vi "generate_DAC_voltages_V3_justMineZtrajectory.vi"(7 "focus mode?":bool, 8 "derived values":T1, 9 "scan specification":T4={"x amplitude"=0, "x resolution (pixels)"=0, "x offset fly-forward (iterations)"=0, "x offset fly-back (iterations)"=0, "y resolution (nr. of lines)"=0, "y step size"=0, "iterations per pixel"=0, "number of frames"=0, "y offset (pixels)"=0, "number of y-brake lines  (before y-fly-back)"=0, "number y-brake lines (after y-fly-back)"=0, "number of y-fly-back steps"=8, "lines per z step"=0, "number of z/intensity tuples"=0, "number of repetitions (volumes or planes)"=0, "z step size derived"=0, "choose the beginning of z scan"=FALSE, "number of frames (settings)"=0, "FPGA trajectory?"=FALSE}, 10 "counter cluster in":T2, 11 "resonant trigger":bool) -> (0 "acquire?":bool, 1 "fly-back acquisition phase?":bool, 2 "counter cluster out":T2, 3 "DAC voltages":T3 {"ch6" max=4095 step=1; "ch5" max=4095 step=1; "ch4" max=4095 step=1; "ch3" max=4095 step=1; "ch2" max=4095 step=1; "ch1" max=4095 step=1; "ch0" max=4095 step=1})   [LabVIEW 2010]
uses:
  scan_specification_cluster.ctl
  common_typedefs/DAC_voltage_cluster.ctl
  counter_cluster.ctl
  derived_values_cluster.ctl
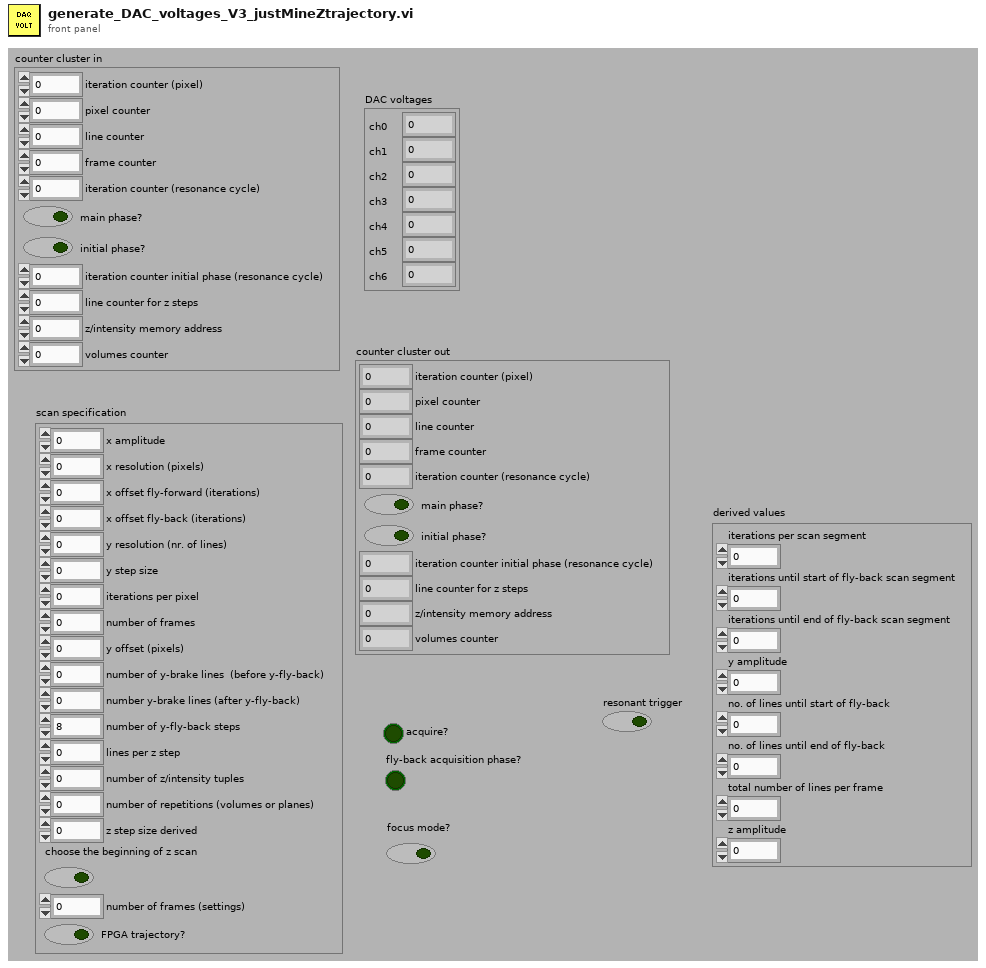
[diagram p1: front panel]
types:
  T1 = typedef "derived_values_cluster.ctl" = cluster{"iterations per scan segment":u16, "iterations until start of fly-back scan segment":u16, "iterations until end of fly-back scan segment":u16, "y amplitude":u16, "no. of lines until start of fly-back":u16, "no. of lines until end of fly-back":u16, "total number of lines per frame ":u16, "z amplitude":u16}
  T2 = typedef "counter_cluster.ctl" = cluster{"iteration counter (pixel)":u16, "pixel counter":u16, "line counter":u16, "frame counter":u16, "iteration counter (resonance cycle)":u16, "main phase?":bool, "initial phase?":bool, "iteration counter initial phase (resonance cycle)":u16, "line counter for z steps":u16, "z/intensity memory address":u32, "volumes counter":u16}
  T3 = typedef "DAC_voltage_cluster.ctl" = cluster{"ch0":u16, "ch1":i16, "ch2":i16, "ch3":u16, "ch4":u16, "ch5":u16, "ch6":u16}
  T4 = typedef "scan_specification_cluster.ctl" = cluster{"x amplitude":u16, "x resolution (pixels)":u16, "x offset fly-forward (iterations)":u16, "x offset fly-back (iterations)":u16, "y resolution (nr. of lines)":u16, "y step size":u16, "iterations per pixel":u16, "number of frames":i32, "y offset (pixels)":u16, "number of y-brake lines  (before y-fly-back)":u16, "number y-brake lines (after y-fly-back)":u16, "number of y-fly-back steps":u16, "lines per z step":u16, "number of z/intensity tuples":u16, "number of repetitions (volumes or planes)":i32, "z step size derived":u16, "choose the beginning of z scan":bool, "number of frames (settings)":i32, "FPGA trajectory?":bool}
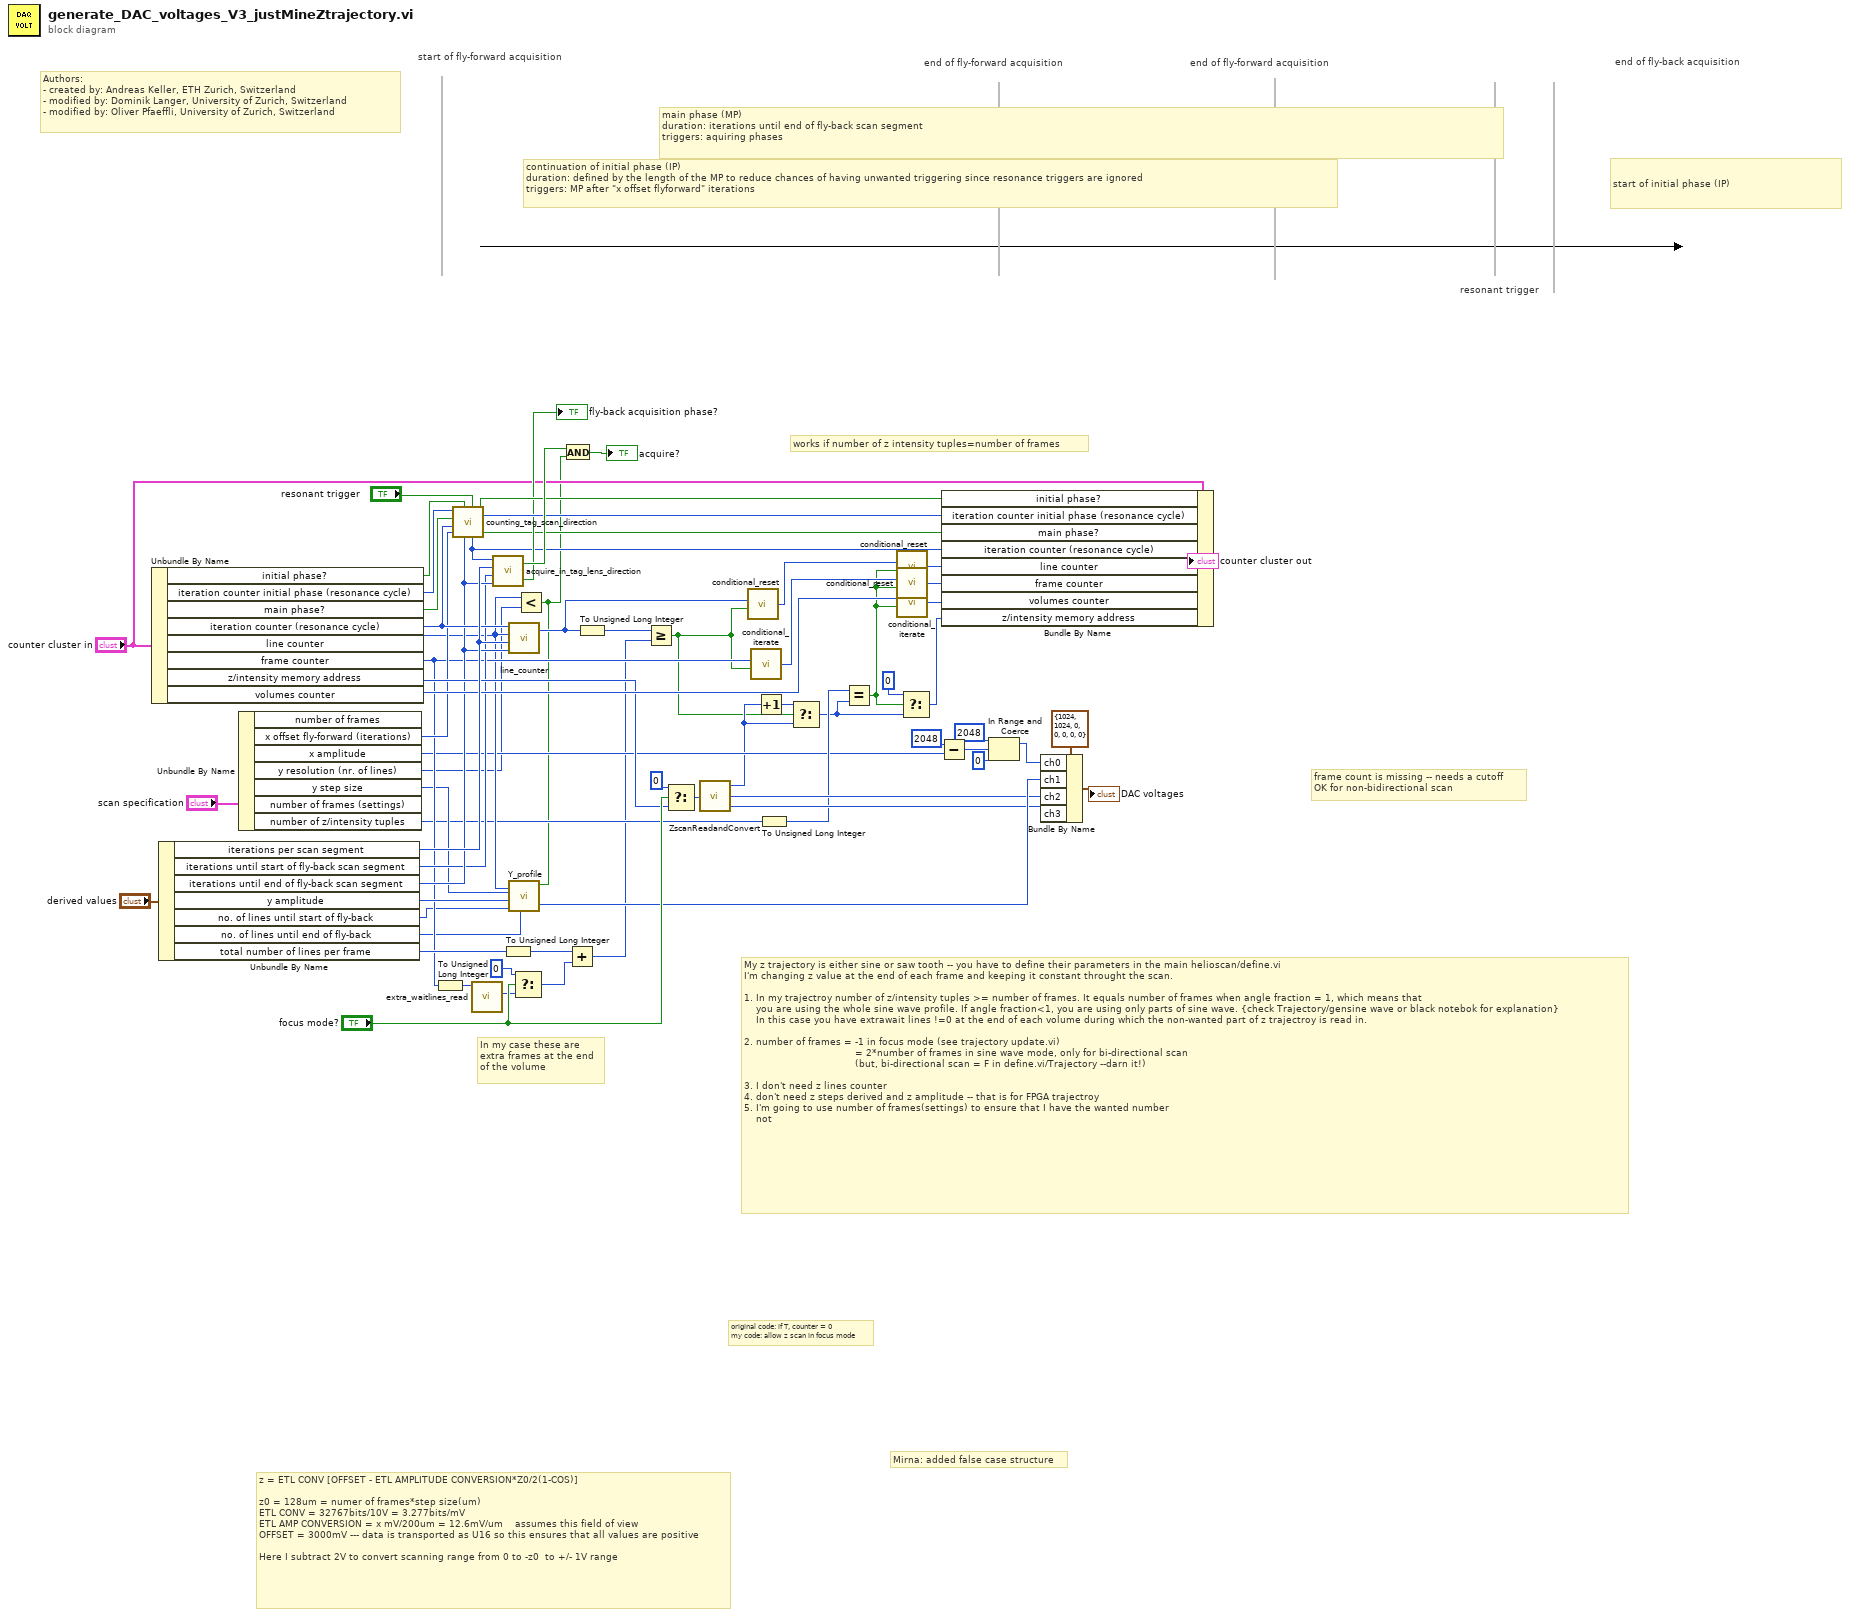
[diagram p0: block diagram]
diagram:
  # "works if number of z intensity tuples=number of frames"
  # "frame count is missing -- needs a cutoff\nOK for non-bidirectional scan"
  # "In my case these are \nextra frames at the end \nof the volume"
  # "My z trajectory is either sine or saw tooth -- you have to define their parameters in the main helioscan/define.vi\nI'm changing z value at the end of each frame and keeping it constant throught the scan.\n\n1. In my trajectroy number of z/intensity tuples >= number of frames. It equals number of frames when angle fraction = 1, which means that \n    you are using the whole sine wave profile. If angle fraction<1, you are using only parts of sine wave. {check Trajectory/gensine wave or black notebok for explanation}\n    In this case you have extrawait lines !=0 at the end of each volume during which the non-wanted part of z trajectroy is read in.\n   \n2. number of frames = -1 in focus mode (see trajectory update.vi)\n                                     = 2*number of frames in sine wave mode, only for bi-directional scan \n                                     (but, bi-directional scan = F in define.vi/Trajectory --darn it!)\n             \n3. I don't need z lines counter\n4. don't need z steps derived and z amplitude -- that is for FPGA trajectroy\n5. I'm going to use number of frames(settings) to ensure that I have the wanted number\n    not"
  # "z = ETL CONV [OFFSET - ETL AMPLITUDE CONVERSION*Z0/2(1-COS)]\n\nz0 = 128um = numer of frames*step size(um)\nETL CONV = 32767bits/10V = 3.277bits/mV\nETL AMP CONVERSION = x mV/200um = 12.6mV/um    assumes this field of view\nOFFSET = 3000mV --- data is transported as U16 so this ensures that all values are positive\n\nHere I subtract 2V to convert scanning range from 0 to -z0  to +/- 1V range"
  # "original code: if T, counter = 0\nmy code: allow z scan in focus mode"
  # "Mirna: added false case structure"
  # "start of initial phase (IP)"
  # "continuation of initial phase (IP)\nduration: defined by the length of the MP to reduce chances of having unwanted triggering since resonance triggers are ignored\ntriggers: MP after \"x offset flyforward\" iterations"
  # "end of fly-back acquisition"
  # "end of fly-forward acquisition"
  # "end of fly-forward acquisition"
  # "start of fly-forward acquisition"
  # "main phase (MP)\nduration: iterations until end of fly-back scan segment\ntriggers: aquiring phases"
  # "resonant trigger"
  # "Authors: \n- created by: Andreas Keller, ETH Zurich, Switzerland\n- modified by: Dominik Langer, University of Zurich, Switzerland\n- modified by: Oliver Pfaeffli, University of Zurich, Switzerland"
  n1 = Unbundle By Name("counter cluster in") -> ("initial phase?"=w56:bool, "iteration counter initial phase (resonance cycle)"=w29:u16, "main phase?"=w47:bool, "iteration counter (resonance cycle)"=w28:u16, "line counter"=w21:u16, "frame counter"=w22:u16, "z/intensity memory address"=w42:u32, "volumes counter"=w49:u16)
  n2 = Unbundle By Name("derived values") -> ("iterations per scan segment"=w55:u16, "iterations until start of fly-back scan segment"=w26:u16, "iterations until end of fly-back scan segment"=w27:u16, "y amplitude"=w33:u16, "no. of lines until start of fly-back"=w19:u16, "no. of lines until end of fly-back"=w18:u16, "total number of lines per frame"=w39:u16)
  n3 = Unbundle By Name("scan specification") -> ("x offset fly-forward (iterations)"=w24:u16, "x amplitude"=w17:u16, "y resolution (nr. of lines)"=w14:u16, "y step size"=w20:u16, "number of z/intensity tuples"=w8:u16)  [unwired: 2 out]
  n4 = To Unsigned Long Integer(number=w22) -> (unsigned 32bit integer=w15:u32)
  n5 = call "counting_tag_scan_direction.vi"("resonant trigger"="resonant trigger", "initial phase?"=w56, "iteration counter initial phase (resonance cycle)"=w29, "main phase?"=w47, "iterations until end of fly-back scan segment"=w27, "iteration counter (resonance cycle)"=w28, "x offset fly-forward (iterations)"=w24) -> ("initial phase? OUT"=w31:bool, "iteration counter initial phase (resonance cycle) out"=w30:u16, "main phase? OUT"=w23:bool, "iteration counter (resonance cycle) out"=w7:u16)
  n6 = call "extra_waitlines_read.vi"("address extra waitlines IN"=w15) -> ("extra waitline data"=w36:u32)  [unwired: 9 in, 1 out]
  n7 = call "acquire_in_tag_lens_direction.vi"("iterations until end of fly-back scan segment"=w27, "iterations until start of fly-back scan segment"=w26, "iterations per scan segment"=w55, "iteration counter (resonance cycle) out"=w7) -> ("flyback phase?"=→"fly-back acquisition phase?":bool, "acquire during flyforward or flyback phase?"=w58:bool)
  n8 = To Unsigned Long Integer(number=w39) -> (unsigned 32bit integer=w38:u32)
  n9 = call "line_counter.vi"("iterations until end of fly-back scan segment"=w27, "iterations per scan segment"=w55, "line counter in"=w21, "iteration counter (resonance cycle)"=w28) -> ("line counter out"=w9:u16)  [unwired: 1 out]
  n10 = Select(t=u32 0, s="focus mode?", f=w36) -> (s? t:f=w2:u32)
  n11 = Less?(x=w21, y=w14) -> (x < y?=w3:bool)
  n12 = call "Y_profile.vi"("no. of lines until end of fly-back"=w18, "line counter"=w21, "no. of lines until start of fly-back"=w19, "y amplitude"=w33, "y step size"=w20, "y acquire? (line counter<number of lines)"=w3) -> ("y signal"=w46:i16)  [unwired: 1 in]
  n13 = And(x=w58, y=w3) -> (x .and. y?=→"acquire?":bool)
  n14 = Add(x=w38, y=w2) -> (x+y=w6:u32)
  n15 = To Unsigned Long Integer(number=w9) -> (unsigned 32bit integer=w37:u32)
  n16 = Greater Or Equal?(x=w37, y=w6) -> (x >= y?=w1:bool)
  n17 = Select(t=u32 0, s="focus mode?", f=w42) -> (s? t:f=w43:u32)
  n18 = call "ZscanReadandConvert.vi"("z/intensity memory address"=w43) -> ("intensity profile"=w45:u16, "z profile"=w44:u16, "address out"=w11:u32)
  n19 = call "conditional_reset.vi"("reset?"=w1, "number in"=w9) -> ("number out"=w52:u16)  [unwired: 4 in]
  n20 = call "conditional_iterate.vi"("iterate?"=w1, "number in"=w22) -> ("number out"=w40:u16)  [unwired: 4 in]
  n21 = Increment(x=w11) -> (x+1=w54:u32)
  n22 = To Unsigned Long Integer(number=w8) -> (unsigned 32bit integer=w35:u32)
  n23 = Select(t=w54, s=w1, f=w11) -> (s? t:f=w4:u32)
  n24 = Equal?(x=w35, y=w4) -> (x = y?=w10:bool)
  n25 = call "conditional_reset.vi"("reset?"=w10, "number in"=w52) -> ("number out"=w51:u16)  [unwired: 4 in]
  n26 = call "conditional_reset.vi"("reset?"=w10, "number in"=w40) -> ("number out"=w41:u16)  [unwired: 4 in]
  n27 = call "conditional_iterate.vi"("iterate?"=w10, "number in"=w49) -> ("number out"=w53:u16)  [unwired: 4 in]
  n28 = Select(t=u32 0, s=w10, f=w4) -> (s? t:f=w12:u32)
  n29 = Subtract(x=u16 2048, y=w17) -> (x-y=w62:u16)
  n30 = Bundle By Name(cluster="counter cluster in", "initial phase?"=w31, "iteration counter initial phase (resonance cycle)"=w30, "main phase?"=w23, "iteration counter (resonance cycle)"=w7, "line counter"=w51, "frame counter"=w41, "volumes counter"=w53, "z/intensity memory address"=w12) -> (→"counter cluster out":T2)
  n31 = In Range and Coerce(upper limit=u16 2048, x=w62, lower limit=u16 0) -> (coerced(x)=w61:u16)  [unwired: 1 out]
  n32 = Bundle By Name(cluster=T3 {"ch0"=1024, "ch1"=1024, "ch2"=0, "ch3"=0, "ch4"=0, "ch5"=0, "ch6"=0} ("DAC voltage"), "ch0"=w61, "ch1"=w46, "ch2"=w44, "ch3"=w45) -> (→"DAC voltages":T3)
